vi "Plotmatrix Plot Page.vi"() -> ()   [LabVIEW 2017, in "XY Plot Matrix.lvclass"]
uses:
  <vilib>/Math Plots/2D Math Plots/XY Plot Matrix/XY Plot Matrix/XY Plot Matrix.lvclass
  <vilib>/Math Plots/2D Math Plots/2D Plot/Action String/XYPlotMatrix Ctrl Act Queue.ctl
  <vilib>/Math Plots/2D Math Plots/2D Plot/Action String/XYPlotMatrix Ctrl Act Cluster.ctl
  <vilib>/Math Plots/2D Math Plots/2D Plot/Action String/2DMathPlot State Class.ctl
  <vilib>/Math Plots/2D Math Plots/XY Plot Matrix/XY Plot Matrix/Typedef/Plotmatrix Property Array.ctl
  <vilib>/Math Plots/2D Math Plots/XY Plot Matrix/XY Plot Matrix/Typedef/Plotmatrix Property.ctl
  <vilib>/Math Plots/2D Math Plots/2D Plot/2D Plot/Typedef/Plot Property Array.ctl
  <vilib>/Math Plots/2D Math Plots/2D Plot/2D Plot/Typedef/Plot Property.ctl
  <vilib>/Math Plots/2D Math Plots/2D Plot/2D Plot/Typedef/Dialog State.ctl
  <vilib>/Math Plots/2D Math Plots/2D Plot/2D Plot/Typedef/Temp Graph State.ctl
  <vilib>/Math Plots/2D Math Plots/2D Plot/2D Plot/Typedef/Temp Graph Property Action.ctl
  <vilib>/Math Plots/2D Math Plots/2D Plot/2D Plot/2D Plot.lvclass
panel:
  out "error out":errorcluster
  in  "Position":i32(ring) items=["(0,0)"]
  in  "Point/fill":u32(colorbox)=16777215
  in  "Interpolation":T1 caption="Plot Interpolation"
  in  "Line Width":T1
  in  "Point Style":T2
  in  "Line Style":T3
  in  "Line":u32(colorbox)
  in  "Active Plot":i32(ring)
  out "Plotmatrix Property Out":T4
  in  "Plotmatrix Property In":T4
  in  "Event Registration":refnum<event-registration>
  in  "Control Ref Queue":T8
  in  "Name":string
  # "Colors"
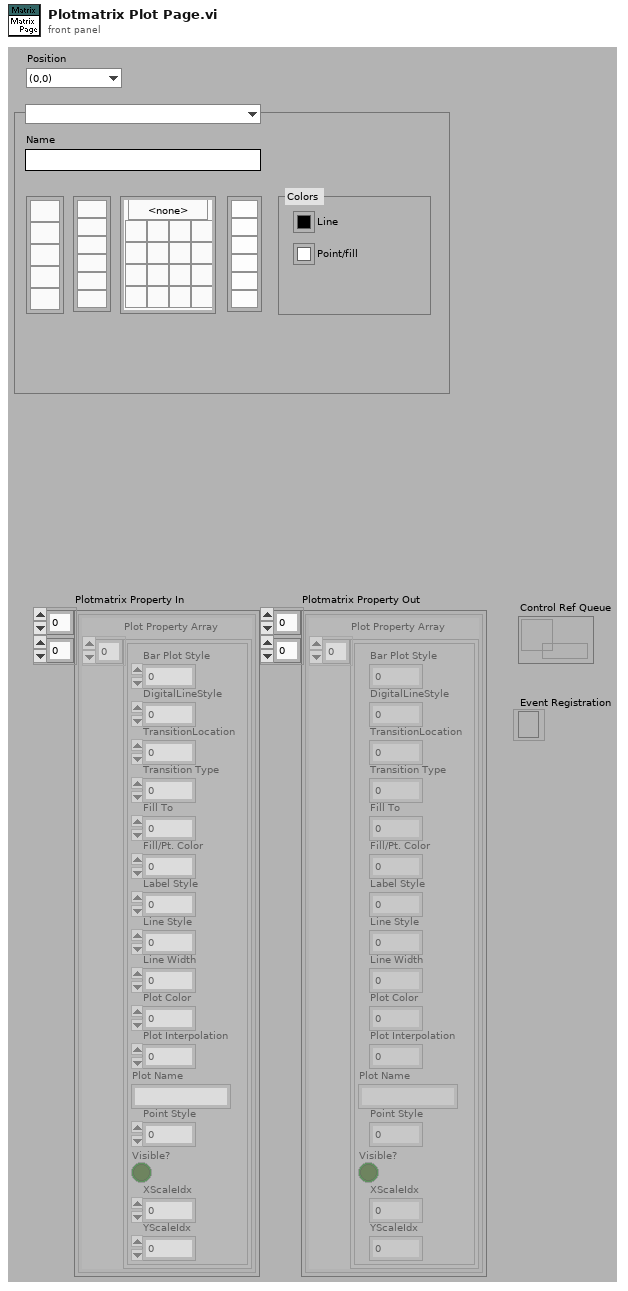
[diagram p1: front panel]
types:
  T1 = cluster{"OK Button 2":bool, "OK Button 3":bool, "OK Button 4":bool, "OK Button 5":bool, "OK Button 6":bool, "OK Button 7":bool}
  T2 = cluster{"OK Button 17":bool, "OK Button":bool, "OK Button 2":bool, "OK Button 3":bool, "OK Button 4":bool, "OK Button 5":bool, "OK Button 6":bool, "OK Button 7":bool, "OK Button 8":bool, "OK Button 9":bool, "OK Button 10":bool, "OK Button 11":bool, "OK Button 12":bool, "OK Button 13":bool, "OK Button 14":bool, "OK Button 15":bool, "OK Button 16":bool}
  T3 = cluster{"OK Button":bool, "OK Button 2":bool, "OK Button 3":bool, "OK Button 4":bool, "OK Button 5":bool}
  T4 = typedef "XY Plot Matrix.lvclass/Plotmatrix Property Array.ctl" = T5[][]
  T5 = typedef "XY Plot Matrix.lvclass/Plotmatrix Property.ctl" = cluster{"Plot Property Array":T6}
  T6 = typedef "2D Plot.lvclass/Plot Property Array.ctl" = T7[]
  T7 = typedef "2D Plot.lvclass/Plot Property.ctl" = cluster{"Bar Plot Style":u8, "DigitalLineStyle":u8, "TransitionLocation":u8, "Transition Type":u8, "Fill To":i16, "Fill/Pt. Color":u32, "Label Style":u8, "Line Style":u8, "Line Width":u8, "Plot Color":u32, "Plot Interpolation":u8, "Plot Name":string, "Point Style":u8, "Visible?":bool, "XScaleIdx":u32, "YScaleIdx":u32}
  T8 = typedef "XYPlotMatrix Ctrl Act Queue.ctl" = refnum<queue>
  T9 = typedef "2D Plot.lvclass/Dialog State.ctl" = enum16{"Initialize", "Read Property", "Write Property", "Idle", "Exit"}
  T10 = typedef "XYPlotMatrix Ctrl Act Cluster.ctl" = cluster{"Facade VI":refnum<vi>, "XControl":refnum<vi>, "Sub Panel":refnum<vi>, "Sub VI":refnum<vi>, "Export Image":refnum<vi>, "Display State Change Class":T11}
  T11 = typedef "2DMathPlot State Class.ctl" = enum16{"Update All (Undo)", "Update General", "Update Appearance", "Update Format", "Update Scale", "Update Marker", "Update Cursor", "None"}
  T12 = typedef "2D Plot.lvclass/Temp Graph Property Action.ctl" = enum16{"Appearance Property", "Format Property", "Plots Property", "Scales Property"}
  T13 = typedef "2D Plot.lvclass/Temp Graph State.ctl" = enum16{"Create", "Update Graph", "Update Property Only", "Get Plot Name", "Get Axis Name", "Destory"}
  T14 = cluster{"Bool Array[0]":bool, "Bool Array[1]":bool, "Bool Array[2]":bool, "Bool Array[3]":bool, "Bool Array[4]":bool}
  T15 = cluster{"Bool Array[0]":bool, "Bool Array[1]":bool, "Bool Array[2]":bool, "Bool Array[3]":bool, "Bool Array[4]":bool, "Bool Array[5]":bool}
  T16 = cluster{"Bool Array[0]":bool, "Bool Array[1]":bool, "Bool Array[2]":bool, "Bool Array[3]":bool, "Bool Array[4]":bool, "Bool Array[5]":bool, "Bool Array[6]":bool, "Bool Array[7]":bool, "Bool Array[8]":bool, "Bool Array[9]":bool, "Bool Array[10]":bool, "Bool Array[11]":bool, "Bool Array[12]":bool, "Bool Array[13]":bool, "Bool Array[14]":bool, "Bool Array[15]":bool, "Bool Array[16]":bool}
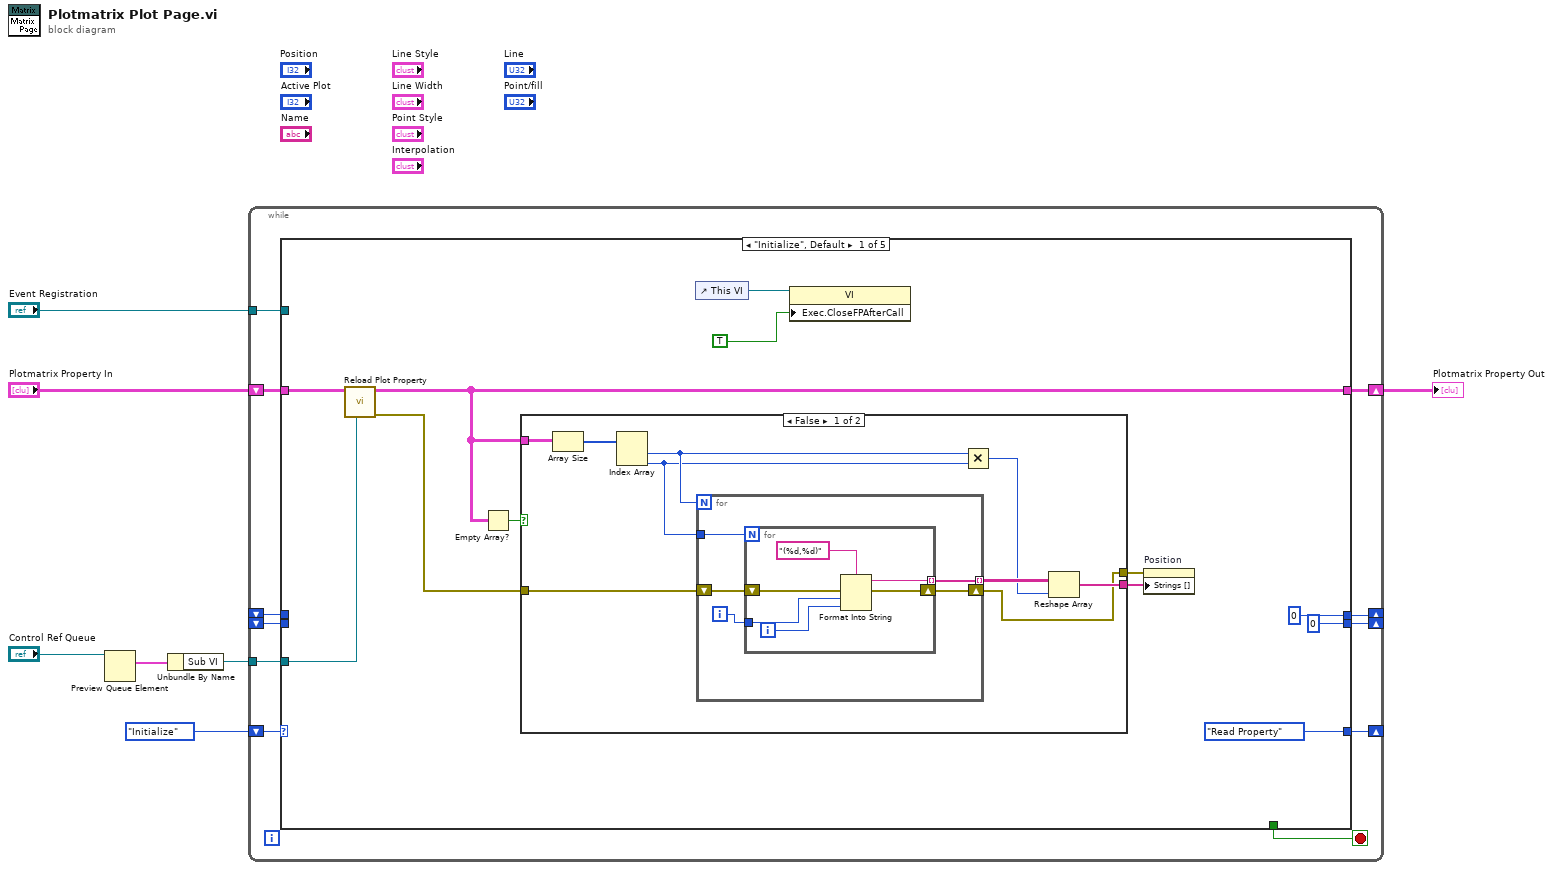
[diagram p0: block diagram]
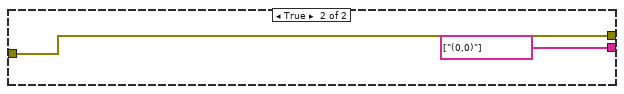
[diagram p2: hidden frame]
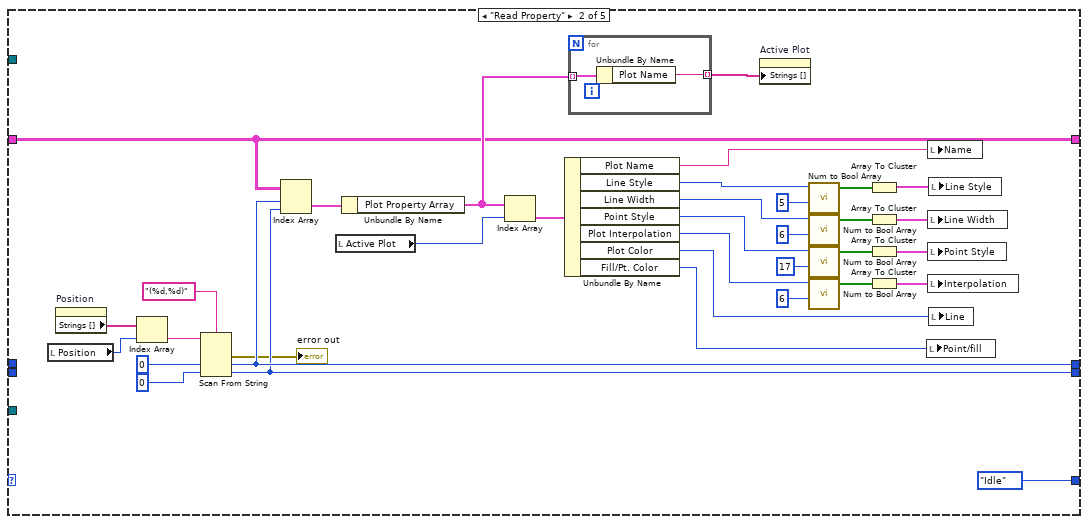
[diagram p3: hidden frame]
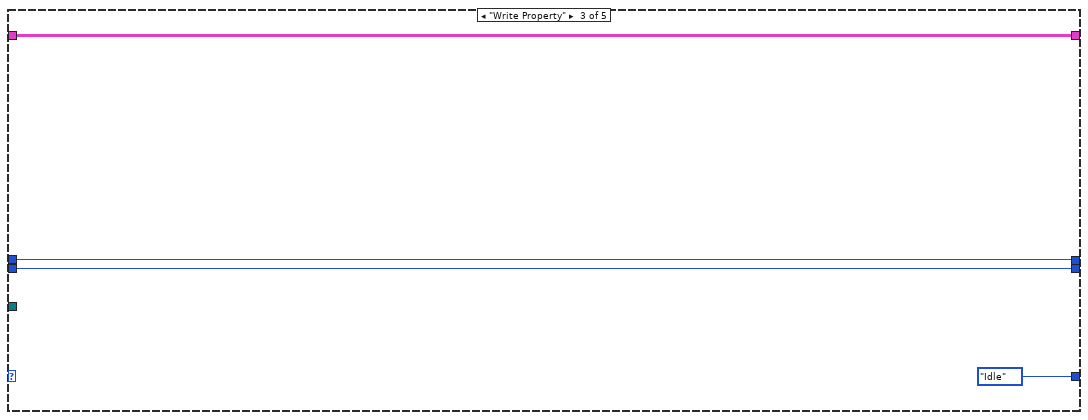
[diagram p4: hidden frame]
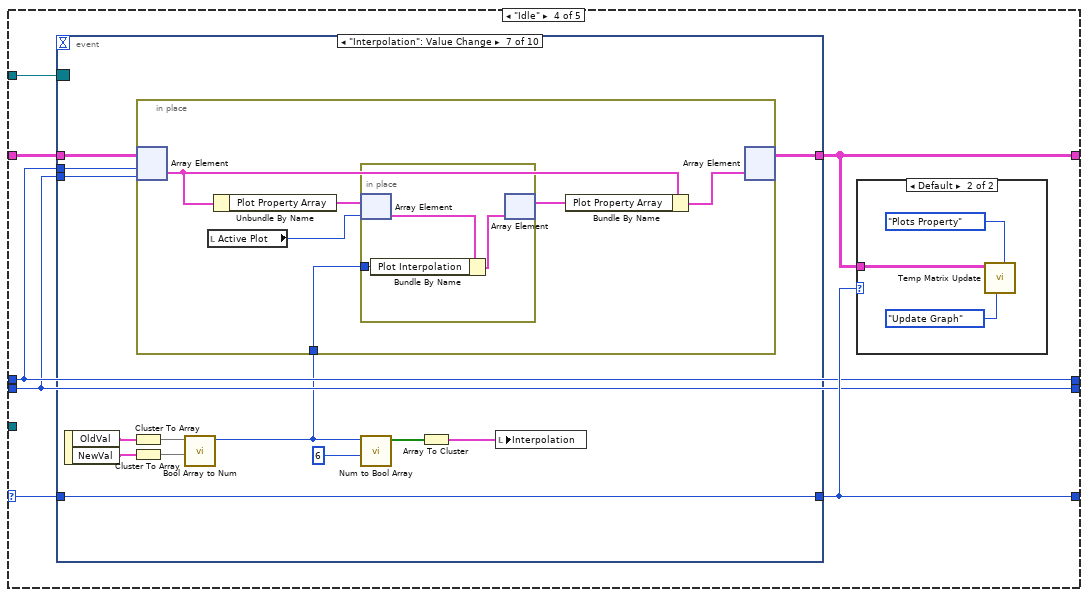
[diagram p5: hidden frame]
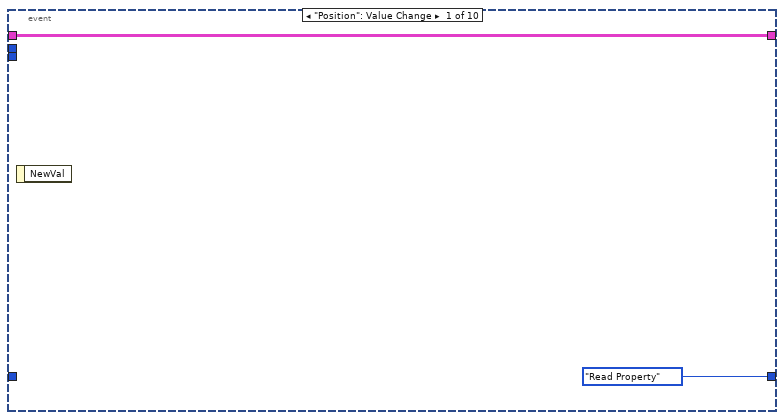
[diagram p7: hidden frame]
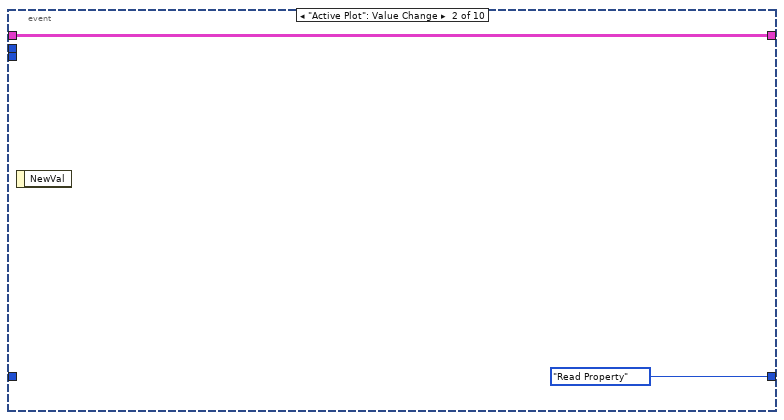
[diagram p8: hidden frame]
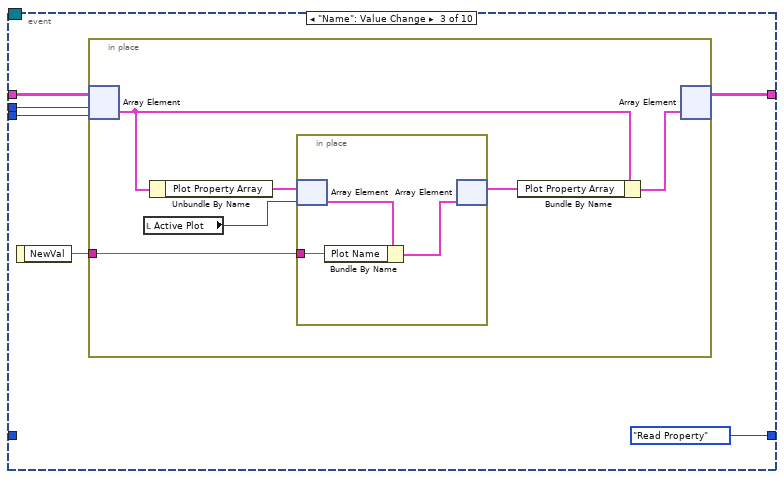
[diagram p9: hidden frame]
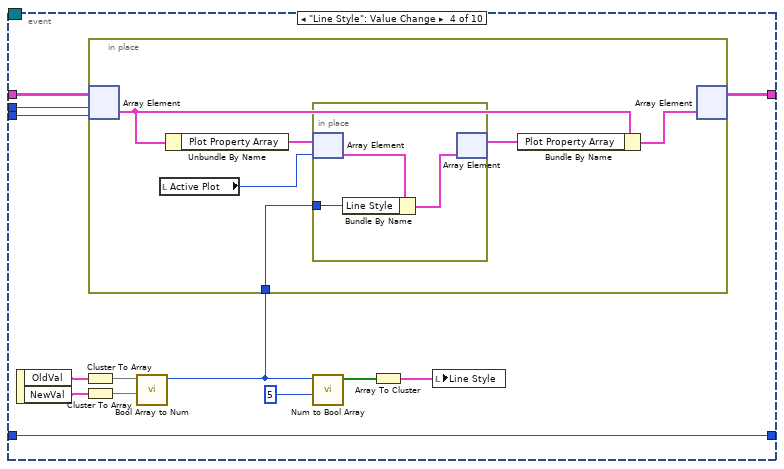
[diagram p10: hidden frame]
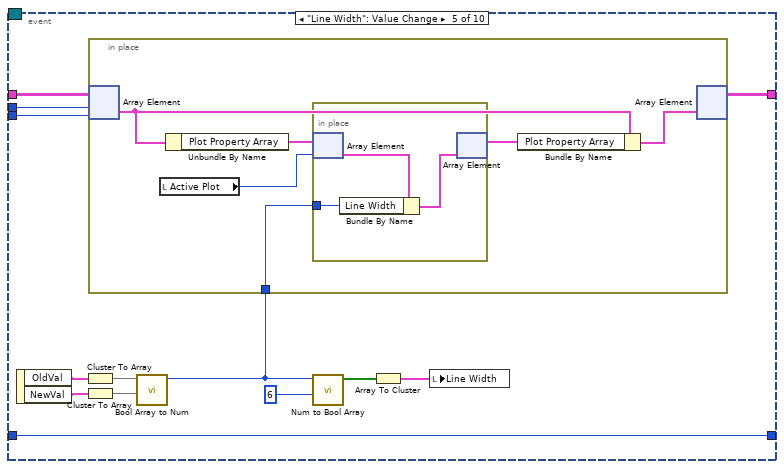
[diagram p11: hidden frame]
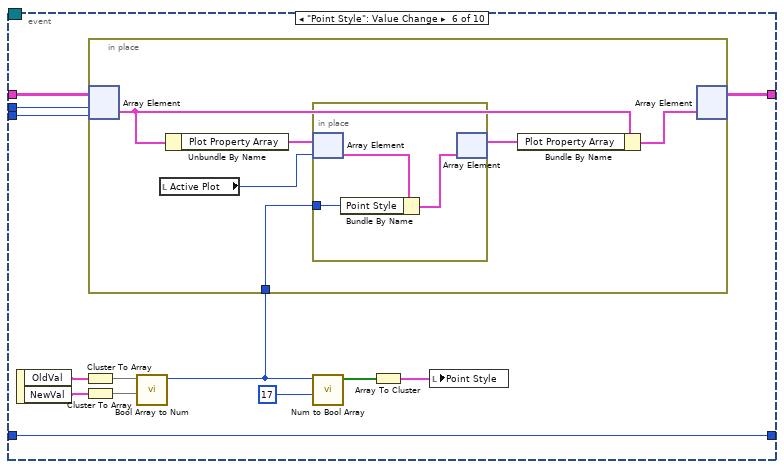
[diagram p12: hidden frame]
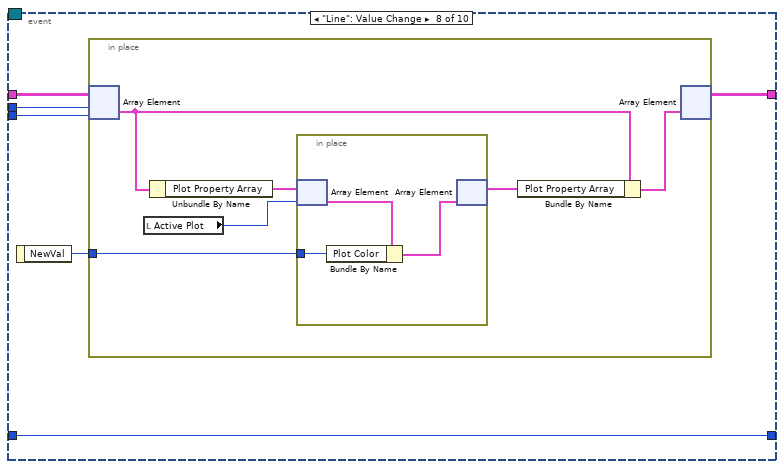
[diagram p13: hidden frame]
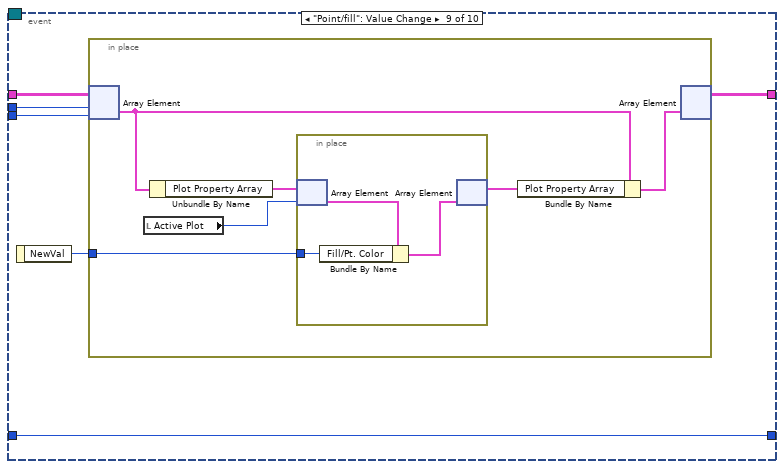
[diagram p14: hidden frame]
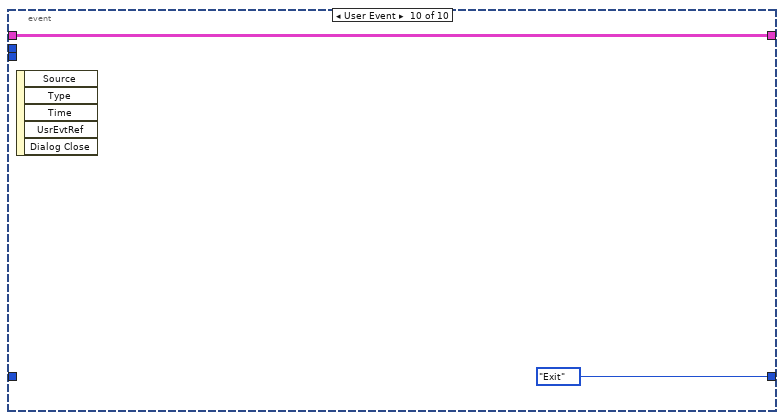
[diagram p15: hidden frame]
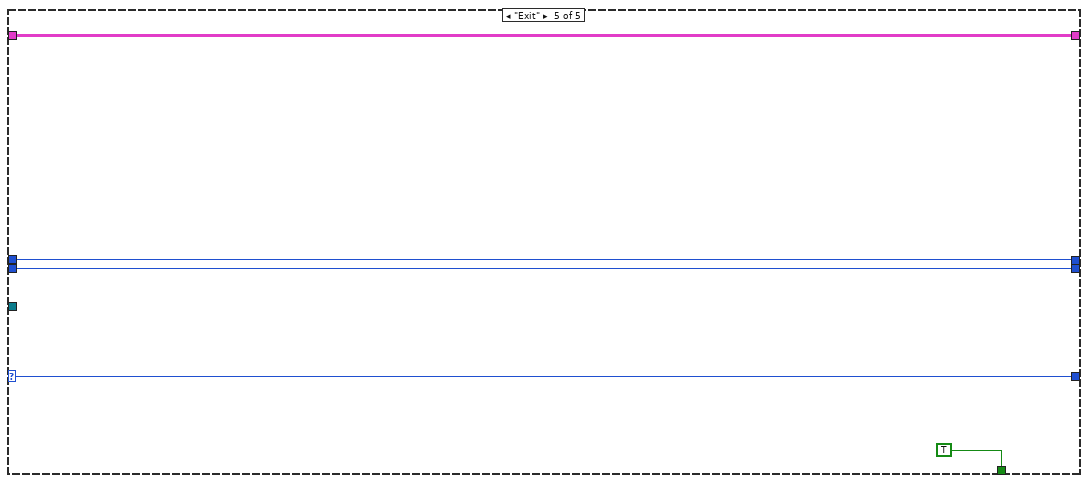
[diagram p16: hidden frame]
diagram:
  n1 = Preview Queue Element(queue="Control Ref Queue") -> (element=w2:T10)  [unwired: 1 in, 4 out]
  n2 = Unbundle By Name(w2) -> ("Sub VI"=w1:refnum<vi>)
  n3 = while {
    tunnel: "Event Registration" -> [w17]
    shift-right: [w14] -> _
    shift-left: Dialog_State."Initialize" ("Enum") -> [w18]
    shift-right: [w15] -> w4
    shift-left: "Plotmatrix Property In" -> [w16]
    shift-right: [w12] -> _
    shift-left: _ -> [w10]
    shift-right: [w11] -> _
    shift-left: _ -> [w9]
    tunnel: w1 -> [w8]
    stop <- w13 stop-if-true
    n4 = case shown="\"Initialize\", Default" w18 {
      selector: w18 -> [_ _ _ w98 w247]
      tunnel: w17 -> [_ _ _ w100 _]
      tunnel: w16 -> [w27 w67 w92 w99 w245]
      tunnel: [w20 w67 w92 w97 w245] -> w15
      tunnel: [Dialog_State."Read Property" ("Enum") Dialog_State."Idle" ("Enum") Dialog_State."Idle" ("Enum") w96 w247] -> w14
      tunnel: [_ _ _ _ TRUE] -> w13
      tunnel: [0 ("default value 1") w55 w91 w95 w244] -> w12
      tunnel: [0 ("default value 2") w54 w90 w94 w243] -> w11
      tunnel: w10 -> [_ _ w91 w95 w244]
      tunnel: w9 -> [_ _ w90 w94 w243]
      tunnel: w8 -> [w23 _ _ _ _]
      frame "Initialize", Default {
        n5 = call <vilib>:"Reload Plot Property.vi"("Sub VI"=w23, "Plot Property Array In"=w27) -> ("error out"=w22:errorcluster, "Plot Property Array Out"=w20:T4)  [unwired: 1 in, 7 out]
        n6 = Empty Array?(array=w20) -> (empty?=w19:bool)
        n7 = case shown="False" w19 {
          tunnel: [w38 string[] ["(0,0)"]] -> w26
          tunnel: w20 -> [w37 _]
          tunnel: w22 -> [w32 w52]
          tunnel: [w31 w52] -> w21
          frame False {
            n8 = Array Size(array=w37) -> (size(s)=w36:i32[])
            n9 = Index Array(array=w36) -> (element #1=w35:i32, element #2=w34:i32)  [unwired: 2 in]
            n10 = for {
              N: w35 -> [_]
              tunnel: [w44] -> w39 mode=indexing
              tunnel: w34 -> [w42]
              shift-right: [w40] -> w31
              shift-left: w32 -> [w41]
              i -> [w43]
              n11 = for {
                N: w42 -> [_]
                tunnel: w43 -> [w50]
                tunnel: [w48] -> w44 mode=indexing
                shift-right: [w45] -> w40
                shift-left: w41 -> [w46]
                i -> [w47]
                n12 = Format Into String(format string="(%d,%d)", error in=w46, w50, w47) -> (resulting string=w48:string, error out=w45:errorcluster)  [unwired: 1 in]
              }
            }
            n13 = Multiply(x=w35, y=w34) -> (x*y=w33:i32)
            n14 = Reshape Array(w39, w33) -> (w38:string[])
          }
          frame True {
          }
        }
        n15 = control-ref of="This VI"() -> (w29:refnum<vi>)
        n16 = property class="VI"(reference=w29, "Exec.CloseFPAfterCall"=TRUE ("Execution:Close After Call")) -> ()  [unwired: 1 in, 2 out]
        n17 = property on="Position" class="Ring (strict)"(error in=w21, "Strings []"=w26) -> ()  [unwired: 1 in, 2 out]
      }
      frame "Read Property" {
        n18 = local read "Position"() -> (w72:i32)
        n19 = property on="Position" class="Ring (strict)"() -> ("Strings []"=w73:string[])  [unwired: 2 in, 2 out]
        n20 = Index Array(array=w73, index=w72) -> (element=w71:string)
        n21 = Scan From String(format string="(%d,%d)", input string=w71, default 1=0 ("default value 1"), default 2=0 ("default value 2")) -> (error out=→"error out":errorcluster, output 1=w55:i32, output 2=w54:i32)  [unwired: 2 in, 2 out]
        n22 = Index Array(array=w67, index (row)=w55, index (col)=w54) -> (element=w66:T5)
        n23 = local read "Active Plot"() -> (w87:i32)
        n24 = Unbundle By Name(w66) -> ("Plot Property Array"=w75:T6)
        n25 = Index Array(array=w75, index=w87) -> (element=w86:T7)
        n26 = Unbundle By Name(w86) -> ("Plot Name"=w85:string, "Line Style"=w84:u8, "Line Width"=w77:u8, "Point Style"=w62:u8, "Plot Interpolation"=w58:u8, "Plot Color"=w57:u32, "Fill/Pt. Color"=w56:u32)
        n27 = for {
          tunnel: w75 -> [w89] mode=indexing
          tunnel: [w88] -> w74 mode=indexing
          n28 = Unbundle By Name(w89) -> ("Plot Name"=w88:string)
        }
        n29 = property on="Active Plot" class="Ring (strict)"("Strings []"=w74) -> ()  [unwired: 2 in, 2 out]
        n30 = call <vilib>:"Num to Bool Array.vi"("Array Size"=5, "Value"=w84) -> ("Bool Array"=w82:bool[])  [unwired: 9 out]
        n31 = call <vilib>:"Num to Bool Array.vi"("Array Size"=6, "Value"=w77) -> ("Bool Array"=w80:bool[])  [unwired: 9 out]
        n32 = call <vilib>:"Num to Bool Array.vi"("Array Size"=17, "Value"=w62) -> ("Bool Array"=w64:bool[])  [unwired: 9 out]
        n33 = call <vilib>:"Num to Bool Array.vi"("Array Size"=6, "Value"=w58) -> ("Bool Array"=w60:bool[])  [unwired: 9 out]
        n34 = Array To Cluster(array=w82) -> (cluster=w81:T14)
        n35 = Array To Cluster(array=w80) -> (cluster=w78:T15)
        n36 = Array To Cluster(array=w64) -> (cluster=w63:T16)
        n37 = Array To Cluster(array=w60) -> (cluster=w59:T15)
        n38 = local write "Point/fill"(w56) -> ()
        n39 = local write "Name"(w85) -> ()
        n40 = local write "Line Width"(w78) -> ()
        n41 = local write "Point Style"(w63) -> ()
        n42 = local write "Interpolation"(w59) -> ()
        n43 = local write "Line Style"(w81) -> ()
        n44 = local write "Line"(w57) -> ()
      }
      frame "Write Property" {
      }
      frame "Idle" {
        n45 = event shown="[6] \"Interpolation\": Value Change" {
          selector: w100 -> [_ _ _ _ _ _ _ _ _ _]
          dyn-events: _ -> [_ _ _ _ _ _ _ _ _ _]
          timeout: _ -> [_ _ _ _ _ _ _ _ _ _]
          tunnel: w99 -> [w105 w107 w111 w126 w148 w170 w192 w215 w230 w241]
          tunnel: [w105 w107 w110 w123 w145 w167 w189 w214 w229 w241] -> w97
          tunnel: [Dialog_State."Read Property" ("Enum") Dialog_State."Read Property" ("Enum") Dialog_State."Read Property" ("Enum") w127 w149 w171 w193 w211 w226 Dialog_State."Exit" ("Enum")] -> w96
          tunnel: w98 -> [_ _ _ w127 w149 w171 w193 w211 w226 _]
          tunnel: w95 -> [_ _ w109 w125 w147 w169 w191 w213 w228 _]
          tunnel: w94 -> [_ _ w108 w124 w146 w168 w190 w212 w227 _]
          event "Position": Value Change {
            n46 = event-data() -> ()  [unwired: 2 out]
          }
          event "Active Plot": Value Change {
            n47 = event-data() -> ()  [unwired: 2 out]
          }
          event "Name": Value Change {
            n48 = event-data() -> ("NewVal"=w113:string)  [unwired: 1 out]
            n49 = in-place {
              in-place-border: w113 -> [w119]
              n50 = in-place-array #1(w111, w109, w108) -> (w118:T5)
              n51 = local read "Active Plot"() -> (w114:i32)
              n52 = Unbundle By Name(w118) -> ("Plot Property Array"=w115:T6)
              n53 = in-place {
                in-place-border: w119 -> [w120]
                n54 = in-place-array #2(w115, w114) -> (w122:T7)
                n55 = Bundle By Name(cluster=w122, "Plot Name"=w120) -> (w121:T7)
                n56 = in-place-array #2(w121) -> (w116:T6)  [unwired: 1 out]
              }
              n57 = Bundle By Name(cluster=w118, "Plot Property Array"=w116) -> (w117:T5)
              n58 = in-place-array #1(w117) -> (w110:T4)  [unwired: 2 out]
            }
          }
          event "Line Style": Value Change {
            n59 = event-data() -> ("OldVal"=w131:T3, "NewVal"=w130:T3)  [unwired: 1 out]
            n60 = Cluster To Array(cluster=w131) -> (array=w133:bool[])
            n61 = Cluster To Array(cluster=w130) -> (array=w132:bool[])
            n62 = call <vilib>:"Bool Array to Num.vi"("New Bool Array"=w132, "Old Bool Array"=w133) -> ("Value"=w128:u8)  [unwired: 9 out]
            n63 = in-place {
              in-place-border: w128 -> [w138]
              n64 = in-place-array #3(w126, w125, w124) -> (w137:T5)
              n65 = local read "Active Plot"() -> (w140:i32)
              n66 = Unbundle By Name(w137) -> ("Plot Property Array"=w141:T6)
              n67 = in-place {
                in-place-border: w138 -> [w142]
                n68 = in-place-array #4(w141, w140) -> (w144:T7)
                n69 = Bundle By Name(cluster=w144, "Line Style"=w142) -> (w143:T7)
                n70 = in-place-array #4(w143) -> (w139:T6)  [unwired: 1 out]
              }
              n71 = Bundle By Name(cluster=w137, "Plot Property Array"=w139) -> (w136:T5)
              n72 = in-place-array #3(w136) -> (w123:T4)  [unwired: 2 out]
            }
            n73 = call <vilib>:"Num to Bool Array.vi"("Array Size"=5, "Value"=w128) -> ("Bool Array"=w135:bool[])  [unwired: 9 out]
            n74 = Array To Cluster(array=w135) -> (cluster=w129:T14)
            n75 = local write "Line Style"(w129) -> ()
          }
          event "Line Width": Value Change {
            n76 = event-data() -> ("OldVal"=w153:T1, "NewVal"=w152:T1)  [unwired: 1 out]
            n77 = Cluster To Array(cluster=w153) -> (array=w155:bool[])
            n78 = Cluster To Array(cluster=w152) -> (array=w154:bool[])
            n79 = call <vilib>:"Bool Array to Num.vi"("New Bool Array"=w154, "Old Bool Array"=w155) -> ("Value"=w150:u8)  [unwired: 9 out]
            n80 = in-place {
              in-place-border: w150 -> [w160]
              n81 = in-place-array #5(w148, w147, w146) -> (w159:T5)
              n82 = local read "Active Plot"() -> (w162:i32)
              n83 = Unbundle By Name(w159) -> ("Plot Property Array"=w163:T6)
              n84 = in-place {
                in-place-border: w160 -> [w164]
                n85 = in-place-array #6(w163, w162) -> (w166:T7)
                n86 = Bundle By Name(cluster=w166, "Line Width"=w164) -> (w165:T7)
                n87 = in-place-array #6(w165) -> (w161:T6)  [unwired: 1 out]
              }
              n88 = Bundle By Name(cluster=w159, "Plot Property Array"=w161) -> (w158:T5)
              n89 = in-place-array #5(w158) -> (w145:T4)  [unwired: 2 out]
            }
            n90 = call <vilib>:"Num to Bool Array.vi"("Array Size"=6, "Value"=w150) -> ("Bool Array"=w157:bool[])  [unwired: 9 out]
            n91 = Array To Cluster(array=w157) -> (cluster=w151:T15)
            n92 = local write "Line Width"(w151) -> ()
          }
          event "Point Style": Value Change {
            n93 = event-data() -> ("OldVal"=w175:T2, "NewVal"=w174:T2)  [unwired: 1 out]
            n94 = Cluster To Array(cluster=w175) -> (array=w177:bool[])
            n95 = Cluster To Array(cluster=w174) -> (array=w176:bool[])
            n96 = call <vilib>:"Bool Array to Num.vi"("New Bool Array"=w176, "Old Bool Array"=w177) -> ("Value"=w172:u8)  [unwired: 9 out]
            n97 = in-place {
              in-place-border: w172 -> [w182]
              n98 = in-place-array #7(w170, w169, w168) -> (w181:T5)
              n99 = local read "Active Plot"() -> (w184:i32)
              n100 = Unbundle By Name(w181) -> ("Plot Property Array"=w185:T6)
              n101 = in-place {
                in-place-border: w182 -> [w186]
                n102 = in-place-array #8(w185, w184) -> (w188:T7)
                n103 = Bundle By Name(cluster=w188, "Point Style"=w186) -> (w187:T7)
                n104 = in-place-array #8(w187) -> (w183:T6)  [unwired: 1 out]
              }
              n105 = Bundle By Name(cluster=w181, "Plot Property Array"=w183) -> (w180:T5)
              n106 = in-place-array #7(w180) -> (w167:T4)  [unwired: 2 out]
            }
            n107 = call <vilib>:"Num to Bool Array.vi"("Array Size"=17, "Value"=w172) -> ("Bool Array"=w179:bool[])  [unwired: 9 out]
            n108 = Array To Cluster(array=w179) -> (cluster=w173:T16)
            n109 = local write "Point Style"(w173) -> ()
          }
          event "Interpolation": Value Change {
            n110 = event-data() -> ("OldVal"=w197:T1, "NewVal"=w196:T1)  [unwired: 1 out]
            n111 = Cluster To Array(cluster=w197) -> (array=w199:bool[])
            n112 = Cluster To Array(cluster=w196) -> (array=w198:bool[])
            n113 = call <vilib>:"Bool Array to Num.vi"("New Bool Array"=w198, "Old Bool Array"=w199) -> ("Value"=w194:u8)  [unwired: 9 out]
            n114 = in-place {
              in-place-border: w194 -> [w204]
              n115 = in-place-array #9(w192, w191, w190) -> (w203:T5)
              n116 = local read "Active Plot"() -> (w206:i32)
              n117 = Unbundle By Name(w203) -> ("Plot Property Array"=w207:T6)
              n118 = in-place {
                in-place-border: w204 -> [w208]
                n119 = in-place-array #10(w207, w206) -> (w210:T7)
                n120 = Bundle By Name(cluster=w210, "Plot Interpolation"=w208) -> (w209:T7)
                n121 = in-place-array #10(w209) -> (w205:T6)  [unwired: 1 out]
              }
              n122 = Bundle By Name(cluster=w203, "Plot Property Array"=w205) -> (w202:T5)
              n123 = in-place-array #9(w202) -> (w189:T4)  [unwired: 2 out]
            }
            n124 = call <vilib>:"Num to Bool Array.vi"("Array Size"=6, "Value"=w194) -> ("Bool Array"=w201:bool[])  [unwired: 9 out]
            n125 = Array To Cluster(array=w201) -> (cluster=w195:T15)
            n126 = local write "Interpolation"(w195) -> ()
          }
          event "Line": Value Change {
            n127 = event-data() -> ("NewVal"=w216:u32)  [unwired: 1 out]
            n128 = in-place {
              in-place-border: w216 -> [w222]
              n129 = in-place-array #11(w215, w213, w212) -> (w221:T5)
              n130 = local read "Active Plot"() -> (w217:i32)
              n131 = Unbundle By Name(w221) -> ("Plot Property Array"=w218:T6)
              n132 = in-place {
                in-place-border: w222 -> [w223]
                n133 = in-place-array #12(w218, w217) -> (w225:T7)
                n134 = Bundle By Name(cluster=w225, "Plot Color"=w223) -> (w224:T7)
                n135 = in-place-array #12(w224) -> (w219:T6)  [unwired: 1 out]
              }
              n136 = Bundle By Name(cluster=w221, "Plot Property Array"=w219) -> (w220:T5)
              n137 = in-place-array #11(w220) -> (w214:T4)  [unwired: 2 out]
            }
          }
          event "Point/fill": Value Change {
            n138 = event-data() -> ("NewVal"=w231:u32)  [unwired: 1 out]
            n139 = in-place {
              in-place-border: w231 -> [w237]
              n140 = in-place-array #13(w230, w228, w227) -> (w236:T5)
              n141 = local read "Active Plot"() -> (w232:i32)
              n142 = Unbundle By Name(w236) -> ("Plot Property Array"=w233:T6)
              n143 = in-place {
                in-place-border: w237 -> [w238]
                n144 = in-place-array #14(w233, w232) -> (w240:T7)
                n145 = Bundle By Name(cluster=w240, "Fill/Pt. Color"=w238) -> (w239:T7)
                n146 = in-place-array #14(w239) -> (w234:T6)  [unwired: 1 out]
              }
              n147 = Bundle By Name(cluster=w236, "Plot Property Array"=w234) -> (w235:T5)
              n148 = in-place-array #13(w235) -> (w229:T4)  [unwired: 2 out]
            }
          }
          event User Event {
            n149 = event-data() -> ()  [unwired: 6 out]
          }
        }
        n150 = case shown="Default" w96 {
          tunnel: w97 -> [_ w103]
          frame "Exit" {
          }
          frame Default {
            n151 = call <vilib>:"Temp Matrix Update.vi"("Property Name"=Temp_Graph_Property_Action."Plots Property", "State"=Temp_Graph_State."Update Graph", "Property In"=w103) -> ()  [unwired: 3 in, 6 out]
          }
        }
      }
      frame "Exit" {
      }
    }
  }
  "Plotmatrix Property Out" <- w4
